vi "Init.vi"(0 "ActionsOnEvents in":refnum<class "ActionsOnEvents.lvclass">, 1 "ActionsClass":string, 2 "Events":T1, 3 "IniFile":path=path "a3s/ini", 5 "error in (no error)":errorcluster) -> (14 "ActionsOnEvents out":refnum<class "ActionsOnEvents.lvclass">, 19 "error out":errorcluster)   [LabVIEW 2017, in "ActionsOnEvents.lvclass"]
uses:
  ActionsOnEvents.lvclass
  SystemEventData/SystemEventsType.ctl
  Actions/ActionBase_class/ActionBase.lvclass
  ActionsOnEvents.lvclass/ActionsOnEvents.ctl
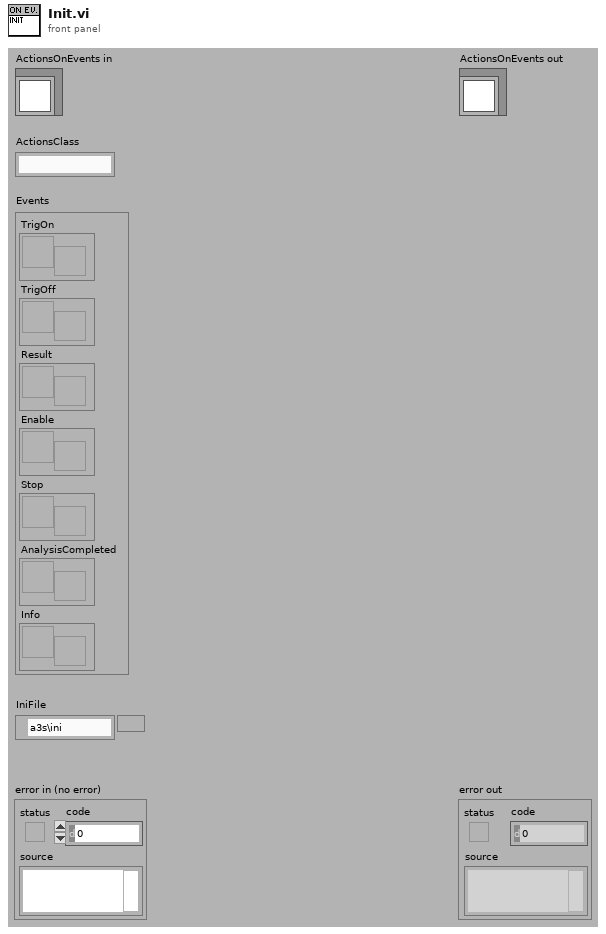
[diagram p1: front panel]
types:
  T1 = typedef "SystemEventsType.ctl" = cluster{"TrigOn":refnum<user-event>, "TrigOff":refnum<user-event>, "Result":refnum<user-event>, "Enable":refnum<user-event>, "Stop":refnum<user-event>, "AnalysisCompleted":refnum<user-event>, "Info":refnum<user-event>}
  T2 = enum32{"invalid app kind", "Development System", "Run Time System", "Student Edition", "Embedded LabVIEW", "Evaluation", "Custom"}
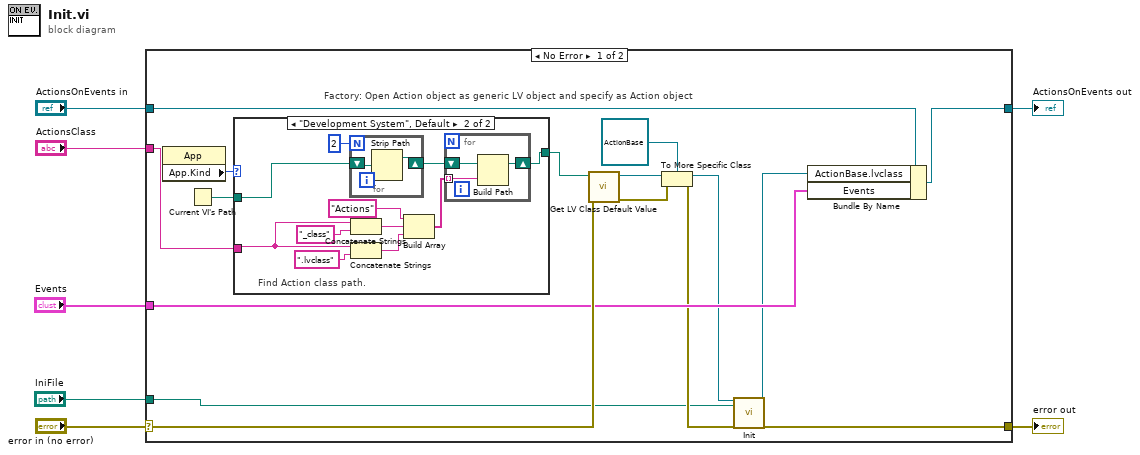
[diagram p0: block diagram]
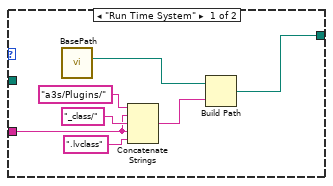
[diagram p2: hidden frame]
diagram:
  n1 = case shown="No Error" "error in (no error)" {
    selector: "error in (no error)" -> [w18 w48]
    tunnel: [w8 w48] -> w6
    tunnel: [w22 w47] -> w4
    tunnel: "ActionsOnEvents in" -> [w23 w47]
    tunnel: "ActionsClass" -> [w16 _]
    tunnel: "Events" -> [w17 _]
    tunnel: "IniFile" -> [w13 _]
    frame No Error {
      # "Factory: Open Action object as generic LV object and specify as Action object"
      n2 = property class="App"() -> ("App.Kind"=w20:T2)  [unwired: 2 in, 2 out]
      n3 = Current VI's Path() -> (path=w11:path)
      n4 = case shown="\"Development System\", Default" w20 {
        tunnel: w16 -> [w26 w38]
        tunnel: [w28 w33] -> w12
        tunnel: w11 -> [_ w31]
        frame "Run Time System" {
          n5 = call "BasePath.vi"() -> ("BasePath"=w24:path)  [unwired: 19 out]
          n6 = Concatenate Strings("a3s/Plugins/" ("name or relative path"), w26, "_class/" ("string"), w26, ".lvclass" ("string")) -> (w29:string)
          n7 = Build Path(base path=w24, name or relative path=w29) -> (appended path=w28:path)
        }
        frame "Development System", Default {
          # "Find Action class path."
          n8 = for {
            N: 2 -> [_]
            shift-right: [w45] -> w41
            shift-left: w31 -> [w46]
            n9 = Strip Path(path=w46) -> (stripped path=w45:path)  [unwired: 1 out]
          }
          n10 = Concatenate Strings(w38, "_class" ("string")) -> (w36:string)
          n11 = Concatenate Strings(w38, ".lvclass" ("string")) -> (w35:string)
          n12 = Build Array("Actions" ("name or relative path"), w36, w35) -> (w34:string[])
          n13 = for {
            shift-right: [w43] -> w33
            shift-left: w41 -> [w44]
            tunnel: w34 -> [w42] mode=indexing
            n14 = Build Path(base path=w44, name or relative path=w42) -> (appended path=w43:path)
          }
        }
      }
      n15 = call <vilib>:"Get LV Class Default Value.vi"("error in (no error)"=w18, "class path"=w12) -> ("error out"=w19:errorcluster, "object"=w10:refnum<class>)  [unwired: 8 out]
      n16 = To More Specific Class(target class=refnum<class "ActionBase.lvclass"> refnum ("ActionBase.lvclass"), reference=w10, error in=w19) -> (specific class reference=w9:refnum<class "ActionBase.lvclass">, error out=w15:errorcluster)
      n17 = call-dynamic "Init.vi"("ActionBase in"=w9, "IniFile"=w13, "error in (no error)"=w15) -> ("ActionBase out"=w14:refnum<class "ActionBase.lvclass">, "error out"=w8:errorcluster)  [unwired: 15 out]
      n18 = Bundle By Name(cluster=w23, "ActionBase.lvclass"=w14, "Events"=w17) -> (w22:refnum<class "ActionsOnEvents.lvclass">)
    }
    frame Error {
    }
  }
  "error out" <- w6
  "ActionsOnEvents out" <- w4
